vi "MUX_example.vi"() -> ()   [LabVIEW 2009]
panel:
  in  "VISA resource name":refnum<visa-resource-name>
  out "Output Results":string[](array[string])
  out "Scan Size":dbl
  out "VISA/Instrument Errors":errorcluster
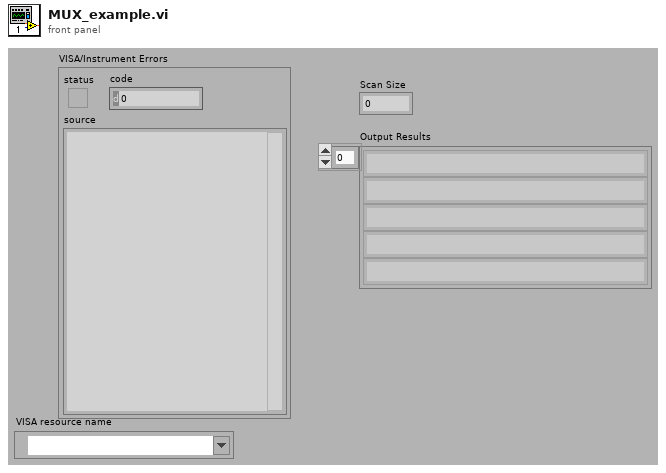
[diagram p1: front panel]
types:
  T1 = enum16{"B-Type", "E-Type", "J-Type", "K-Type", "N-Type", "R-Type", "S-Type", "T-Type"}
  T2 = enum16{"Bus", "Immediate", "External", "Alarm 1", "Alarm 2", "Alarm 3", "Alarm 4", "Timer"}
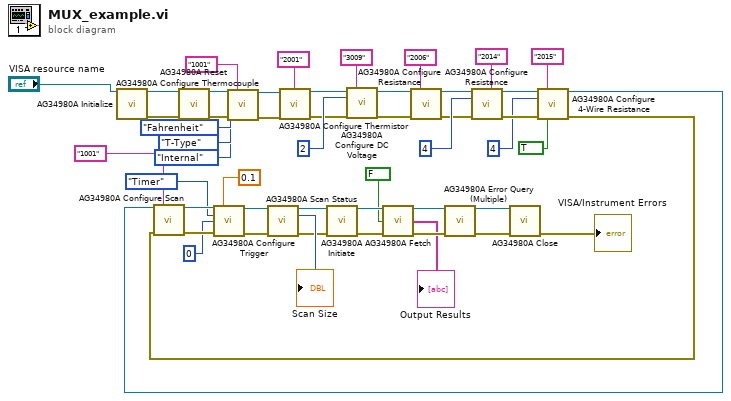
[diagram p0: block diagram]
diagram:
  n1 = call "AG34980A Initialize.vi"("VISA resource name"="VISA resource name") -> ("VISA session"=w50:refnum<visa-resource-name>, "error out"=w49:errorcluster)  [unwired: 13 in]
  n2 = call "AG34980A Reset.vi"("VISA resource name"=w50, "error in (no error)"=w49) -> ("VISA resource name out"=w6:refnum<visa-resource-name>, "error out"=w8:errorcluster)  [unwired: 12 in]
  n3 = call "AG34980A Configure Thermocouple.vi"("VISA resource name"=w6, "Channel List(empty)"="1001", "Reading Units (0:Celcius)"=enum16{"Celcius", "Fahrenheit", "Kelvin"}."Fahrenheit", "Thermocouple Type (2:J-Type)"=T1."T-Type", "Reference Junction Type (2:Fixed)"=enum16{"Internal", "External", "Fixed"}."Internal", "error in (no error)"=w8) -> ("VISA resource name out"=w5:refnum<visa-resource-name>, "error out"=w7:errorcluster)  [unwired: 8 in]
  n4 = call "AG34980A Configure Thermistor.vi"("VISA resource name"=w5, "Channel List(empty)"="2001", "error in (no error)"=w7) -> ("VISA resource name out"=w34:refnum<visa-resource-name>, "error out"=w33:errorcluster)  [unwired: 11 in]
  n5 = call "AG34980A Configure DC Voltage.vi"("VISA resource name"=w34, "Channel List(empty)"="3009", "Range (5:Auto)"=2, "error in (no error)"=w33) -> ("VISA resource name out"=w47:refnum<visa-resource-name>, "error out"=w46:errorcluster)  [unwired: 10 in]
  n6 = call "AG34980A Configure Resistance.vi"("VISA resource name"=w47, "Channel List(empty)"="2006", "error in (no error)"=w46) -> ("VISA resource name out"=w24:refnum<visa-resource-name>, "error out"=w23:errorcluster)  [unwired: 11 in]
  n7 = call "AG34980A Configure Resistance.vi"("VISA resource name"=w24, "Channel List(empty)"="2014", "Range (7:Auto)"=4, "error in (no error)"=w23) -> ("VISA resource name out"=w44:refnum<visa-resource-name>, "error out"=w43:errorcluster)  [unwired: 10 in]
  n8 = call "AG34980A Configure 4-Wire Resistance.vi"("VISA resource name"=w44, "Channel List(empty)"="2015", "Range (7:Auto)"=4, "error in (no error)"=w43, "Offset Compensation (F:Off)"=TRUE) -> ("VISA resource name out"=w39:refnum<visa-resource-name>, "error out"=w40:errorcluster)  [unwired: 9 in]
  n9 = call "AG34980A Configure Scan.vi"("VISA resource name"=w39, "Scan List(empty)"="1001", "error in (no error)"=w40) -> ("VISA resource name out"=w22:refnum<visa-resource-name>, "error out"=w21:errorcluster)  [unwired: 11 in]
  n10 = call "AG34980A Configure Trigger.vi"("VISA resource name"=w22, "Trigger Timer Value (0 sec)"=0.1, "Trigger Source (1:Immediate)"=T2."Timer", "Max Trigger Count (0:Specify Count)"=0, "error in (no error)"=w21) -> ("VISA resource name out"=w31:refnum<visa-resource-name>, "error out"=w30:errorcluster)  [unwired: 9 in]
  n11 = call "AG34980A Scan Status.vi"("VISA resource name"=w31, "error in (no error)"=w30) -> ("VISA resource name out"=w28:refnum<visa-resource-name>, "Scan Size"=→"Scan Size":u32, "error out"=w27:errorcluster)  [unwired: 10 in, 1 out]
  n12 = call "AG34980A Initiate.vi"("VISA resource name"=w28, "error in (no error)"=w27) -> ("VISA resource name out"=w26:refnum<visa-resource-name>, "error out"=w19:errorcluster)  [unwired: 12 in]
  n13 = call "AG34980A Fetch.vi"("VISA resource name"=w26, "Numbers Only (T:On)"=FALSE, "error in (no error)"=w19) -> ("VISA resource name out"=w17:refnum<visa-resource-name>, "Output Data"=→"Output Results":string[], "error out"=w18:errorcluster)  [unwired: 9 in, 1 out]
  n14 = call "AG34980A Error Query (Multiple).vi"("VISA resource name"=w17, "error in (no error)"=w18) -> ("VISA resource name out"=w15:refnum<visa-resource-name>, "error out"=w16:errorcluster)  [unwired: 10 in, 2 out]
  n15 = call "AG34980A Close.vi"("VISA resource name"=w15, "error in (no error)"=w16) -> ("error out"=→"VISA/Instrument Errors":errorcluster)  [unwired: 13 in]
